vi "PLC_Read_REALtest.vi"(4 "addresses":i16[](array[numeric]), 6 "areaType":T1=132 items=["P Area"=128, "I Area"=129, "O Area"=130, "M Area"=131, "DB Area"=132, "Counter Area"=40, "Timer Area"=41], 7 "cpProtocol":i32=122, 8 "Error In":errorcluster, 9 "slot":i32=2, 10 "dataBlock":i32=31, 11 "ip":string="172.18.214.231") -> (0 "Error Out":errorcluster, 2 "results":dbl[](array[numeric]))   [LabVIEW 2014]
uses:
  PLC_Libnodave_wrapper_areaType.ctl
panel:
  out "subarray":u8[](array[numeric])
  out "outBuffer":u8[](array[numeric])
  # "PLC Convert Data (1 REAL - 4 bytes)"
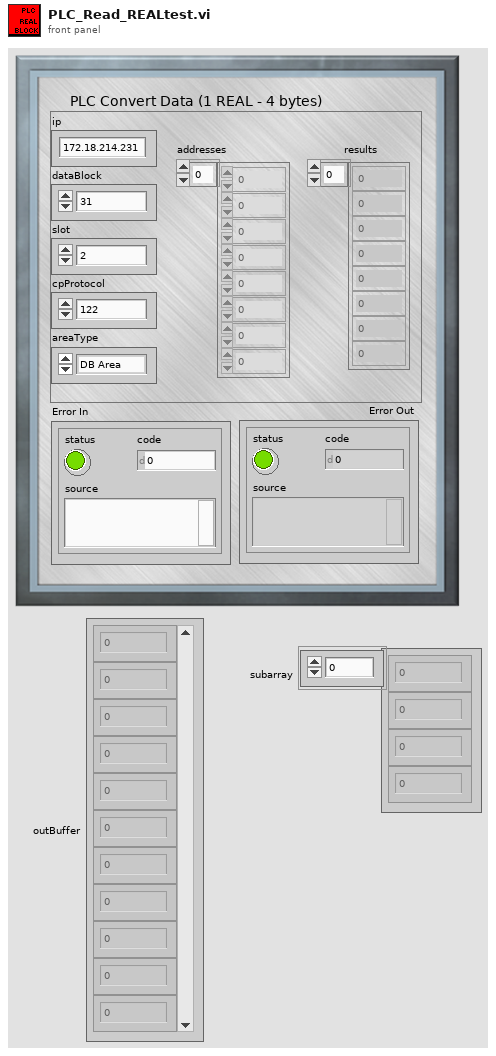
[diagram p1: front panel]
types:
  T1 = typedef "PLC_Libnodave_wrapper_areaType.ctl" = i32
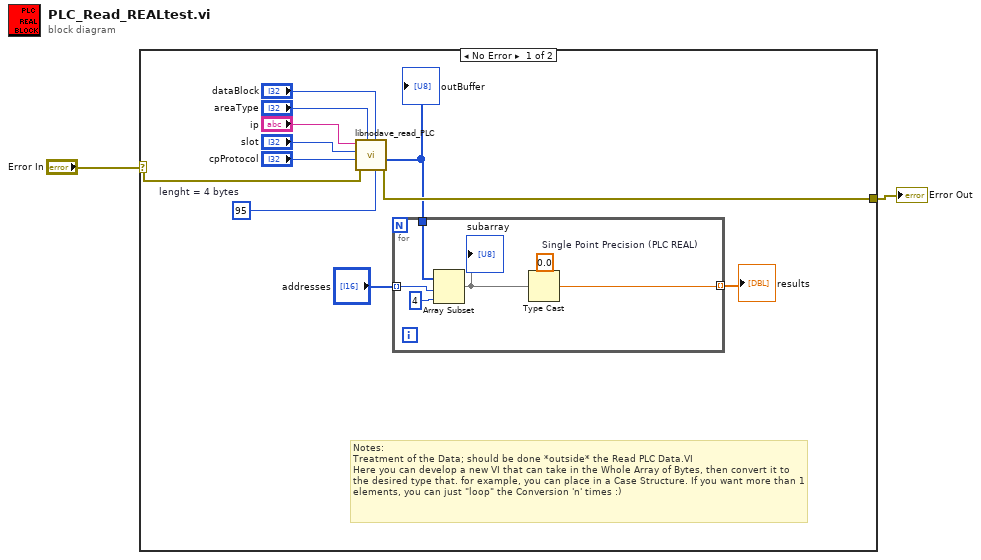
[diagram p0: block diagram]
diagram:
  n1 = case shown="No Error" "Error In" {
    selector: "Error In" -> [w13 w20]
    tunnel: [w12 w20] -> w1
    frame No Error {
      w6 = 95  # lenght = 4 bytes
      # "Notes:\nTreatment of the Data; should be done *outside* the Read PLC Data.VI\nHere you can develop a new VI that can take in the Whole Array of Bytes, then convert it to the desired type that. for example, you can place in a Case Structure. If you want more than 1 elements, you can just \"loop\" the Conversion 'n' times :)"
      n2 = call "libnodave_read_PLC.vi"("length"=w6, "dataBlock"="dataBlock", "areaType"="areaType", "Error In"=w13, "cpProtocol"="cpProtocol", "slot"="slot", "ip"="ip") -> ("Error Out"=w12:errorcluster, "outBuffer"=w5:u8[])  [unwired: 1 in, 2 out]
      "outBuffer" <- w5
      n3 = for {
        tunnel: w5 -> [w18]
        tunnel: [w15] -> w4 mode=indexing
        tunnel: "addresses" -> [w14] mode=indexing
        w19 = sgl 0.0  # Single Point Precision (PLC REAL)
        n4 = Array Subset(array=w18, index=w14, length=4) -> (w16:u8[])
        "subarray" <- w16
        n5 = Type Cast(type=w19, x=w16) -> (*(type *) &x=w15:sgl)
      }
      "results" <- w4
    }
    frame Error {
    }
  }
  "Error Out" <- w1
